vi "PXI-Change AO Gains (by channel).vi"(0 "Multipliers":dbl[](array[numeric]), 5 "Gains":dbl[](array[numeric]), 7 "AO channels":u16[](array[numeric]), 11 "error in (no error)":errorcluster) -> (15 "error out":errorcluster)   [LabVIEW 2015]
doc: "This is a test."
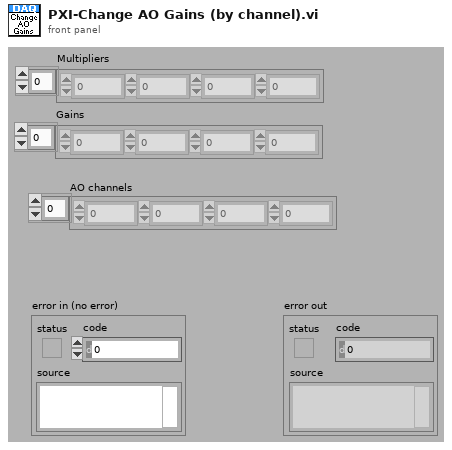
[diagram p1: front panel]
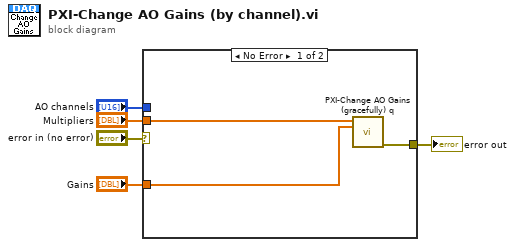
[diagram p0: block diagram]
diagram:
  n1 = case shown="No Error" "error in (no error)" {
    selector: "error in (no error)" -> [_ w9]
    tunnel: "AO channels" -> [_ _]
    tunnel: "Gains" -> [w6 _]
    tunnel: "Multipliers" -> [w7 _]
    tunnel: [w8 w9] -> w1
    frame No Error {
      n2 = call "PXI-Change AO Gains (gracefully) q.vi"("Multipliers in"=w7, "Gains"=w6) -> ("error out"=w8:errorcluster)  [unwired: 13 in]
    }
    frame Error {
    }
  }
  "error out" <- w1
